vi "APC_9049_TS10ms_loop.vi"() -> ()   [LabVIEW 2020]
doc: "This example demonstrates the procedure required to apply different NI-DAQmx Custom Scales to each virtual channel in a task. A DAQmx Task Property Node (Functions >> NI Measurements >> DAQmx - Data Acquisition >> DAQmx Advanced Task Options) is used to obtain the task's virtual channels. A DAQmx Channel Property Node (Functions >> NI Measurements >> DAQmx - Data Acquisition) is then used to set the custom scale for each virtual channel in the task.\n\nThe \"DAQmx Create Scale\" VI creates a custom scale for each channel in the channel list. *Note, make sure your Minimum and Maximum channel parameters are consistent with the range the scale will create."
uses:
  <vilib>/Platform/TimedLoop/XDataNode/timing_clust.ctl
  <vilib>/Platform/TimedLoop/XDataNode/nitl_modes.ctl
  <vilib>/Platform/TimedLoop/XDataNode/wakeup.ctl
  controls/APC_ControlSettings.ctl
  controls/APC_PIDcontrolSettings.ctl
  <vilib>/FPGAPlugInAG/cRIO-9049/niLvFpga_Open_cRIO-9049.vi
  <vilib>/Powertrain Controls/Device Drivers/Tools/Real-Time/Interp1DTableRT.vi
  <vilib>/Utility/error.llb/Error Cluster From Error Code.vi
  <vilib>/rvi/errors/niLvFpgaAdjustHostInterfaceError.vi
  <vilib>/Powertrain Controls/Device Drivers/Tools/Real-Time/time2ticks.vi
  <vilib>/Powertrain Controls/Device Drivers/Tools/Real-Time/Offset2CAT.vi
  <vilib>/FPGAPlugInAG/cRIO-9049/niLvFpga_Close_cRIO-9049.vi
  <vilib>/Platform/TimedLoop/XDataNode/XDataNode.xnode
  <vilib>/rvi/interface/nirviOpenFPGA/nirviOpenFPGA.xnode
  FPGA Bitfiles/nobleapcmulticyl_FPGATarget4_APC9049FPGAmain_30BIM05nubg.lvbitx
  APC_9049_FPGA_main.vi
  <vilib>/rvi/interface/nirviReadWriteControl/nirviReadWriteControl.xnode
  <vilib>/rvi/interface/nirviCloseFPGA/nirviCloseFPGA.xnode
  <vilib>/Platform/TimedLoop/XDataNode/XDNodeRunTimeDep.lvlib
  NiFpgaLv.dll
panel:
  in  "Must Use Cam & Z":bool
  out "FPGA Heartbeat":bool
  in  "manual SA [CADBTDC]":dbl
  in  "manual INJ settings":T1={"Window_Start (DBTDC)"=90.0, "Window_End (DBTDC)"=-30.0, "PilotEnable"=FALSE, "PilotDuration (msec)"=0.0, "PilotAdvance (msec)"=0.0, "PreEnable"=FALSE, "PreDuration (msec)"=0.0, "PreAdvance (msec)"=0.0, "MainEnable"=FALSE, "MainDuration (msec)"=0.0, "MainSOI (DBTDC)"=0.0, "AfterEnable"=FALSE, "AfterDuration (msec)"=0.0, "AfterDelay (msec)"=0.0, "PostEnable"=FALSE, "PostDuration (msec)"=0.0, "PostDelay (msec)"=0.0}
  out "SA [CADBTDC]":dbl format="%.2f"
  in  "Override PC settings":bool
  in  "manual spark enable":bool[](array[boolean])
  in  "manual Injection enable":bool[](array[boolean])
  out "DI_Data Mod6":T2={"ModulePresent"=TRUE, "LVSense"=133, "HVSense"=23, "HVSense2"=1, "TempSense"=33, "Fault1"=126, "Fault2"=0, "OLIntegrator"=0, "HardwareRev"=70, "FirmwareRev"=5}
  in  "PFI0 mode":u8
  out "SparkControl_Out":T3
  in  "1/2 Z pulse":bool=TRUE
  out "toggle TDC":bool
  out "Finished Late? [i-1]":bool
  out "PlsGen_Config_Out":T4={"Channel Enable"=TRUE, "Seq_Start"=10800, "Seq_End"=15600, "Enable_Inj1"=FALSE, "Duration_Inj1"=0, "Timing_Inj1"=0, "Enable_Inj2"=FALSE, "Duration_Inj2"=0, "Timing_Inj2"=0, "Enable_Inj3"=TRUE, "Duration_Inj3"=160000, "Timing_Inj3"=14880, "Enable_Inj4"=FALSE, "Duration_Inj4"=0, "Timing_Inj4"=0, "Enable_Inj5"=FALSE, "Duration_Inj5"=0, "Timing_Inj5"=0}
  out "DI_Data_Mod5":T2={"ModulePresent"=TRUE, "LVSense"=133, "HVSense"=23, "HVSense2"=1, "TempSense"=33, "Fault1"=126, "Fault2"=0, "OLIntegrator"=0, "HardwareRev"=70, "FirmwareRev"=5}
  out "loop time [ms]":u32=10
  out "Speed (RPM)":sgl
  in  "Mod4/DIO7":bool
  in  "Mod4/DIO6":bool
  in  "Mod3/DIO7":bool
  in  "Mod3/DIO6":bool
  in  "Mod3/DIO5":bool
  in  "Mod3/DIO4":bool
  out "InjectionEnable":bool[](array[boolean])=[TRUE, TRUE, TRUE, TRUE, TRUE, TRUE]
  in  "Manual Clear Sync Errors":bool
  out "SparkEnable":bool[](array[boolean])=[TRUE, TRUE, TRUE, TRUE, TRUE, TRUE]
  in  "CutoffPosition (DBTDC)":sgl=-60.0
  out "PlsGen_Time_Config_In":T1={"Window_Start (DBTDC)"=90.0, "Window_End (DBTDC)"=-30.0, "PilotEnable"=FALSE, "PilotDuration (msec)"=0.0, "PilotAdvance (msec)"=0.0, "PreEnable"=FALSE, "PreDuration (msec)"=0.0, "PreAdvance (msec)"=0.0, "MainEnable"=TRUE, "MainDuration (msec)"=4.0, "MainSOI (DBTDC)"=-12.0, "AfterEnable"=FALSE, "AfterDuration (msec)"=0.0, "AfterDelay (msec)"=0.0, "PostEnable"=FALSE, "PostDuration (msec)"=0.0, "PostDelay (msec)"=0.0}
  in  "IPhaseArrayIn":T5(array[cluster])=[{"DriveSrc"=TRUE, "IUpper (A)"=11.0, "ILower (A)"=6.84, "Dur (msec)"=0.35}, {"DriveSrc"=FALSE, "IUpper (A)"=8.0, "ILower (A)"=6.84, "Dur (msec)"=0.25}, {"DriveSrc"=FALSE, "IUpper (A)"=3.9, "ILower (A)"=2.7, "Dur (msec)"=0.0}, {"DriveSrc"=FALSE, "IUpper (A)"=0.0, "ILower (A)"=0.0, "Dur (msec)"=0.0}, {"DriveSrc"=FALSE, "IUpper (A)"=0.0, "ILower (A)"=0.0, "Dur (msec)"=0.0}, {"DriveSrc"=FALSE, "IUpper (A)"=0.0, "ILower (A)"=0.0, "Dur (msec)"=0.0}, {"DriveSrc"=FALSE, "IUpper (A)"=0.0, "ILower (A)"=0.0, "Dur (msec)"=0.0}, {"DriveSrc"=FALSE, "IUpper (A)"=0.0, "ILower (A)"=0.0, "Dur (msec)"=0.0}]
  in  "DIControl":T6={"ModuleEnable"=TRUE, "HVEnable"=FALSE, "InjectEnable"=TRUE, "Phase1FirstPeakEnable"=FALSE, "PiezoEnable"=FALSE, "PiezoInvert"=FALSE, "OneShotSelect"=enum."DISABLED", "One Shot Time (msec)"=1.0, "OneShot"=FALSE, "Fault_ClrSig"=FALSE, "HVTarget (V)"=100.0, "Back Boost Time (msec)"=0.25, "DI Scope Trigger Event"=0, "DI Scope Channel 2"=0} {"DI Scope Trigger Event" items=["INJECTION PULSE", "POWER SUPPLY ENABLED"]; "DI Scope Channel 2" items=["INTERNAL HIGH VOLTAGE", "EXTERNAL HIGH VOLTAGE", "BATTERY VOLTAGE"]}
  in  "EPTControl":T7={"NumberOfCrankTeeth"=3600, "Stroke (FALSE=2, TRUE=4)"=TRUE, "CrankStallPeriod"=5000000, "CrankCountStart"=3600, "PeriodAccumCount"=3600, "SyncEnable"=TRUE, "SimEnable"=FALSE, "MissedCrankFlagClr"=FALSE, "MissedCamFlagClr"=FALSE, "SimPeriod"=500, "WatchdogIn"=FALSE}
  out "EPTData":T8={"CrankSigOS"=FALSE, "CrankStalled"=FALSE, "SyncStopped"=FALSE, "MissedCrankFlag"=FALSE, "MissedCamFlag"=FALSE, "Period"=863, "PeriodAccum"=2084945, "CrankCount"=928, "CurrentPosition"=3712, "MAX_CAT"=28800}
  # "Override PC settings option disabled"
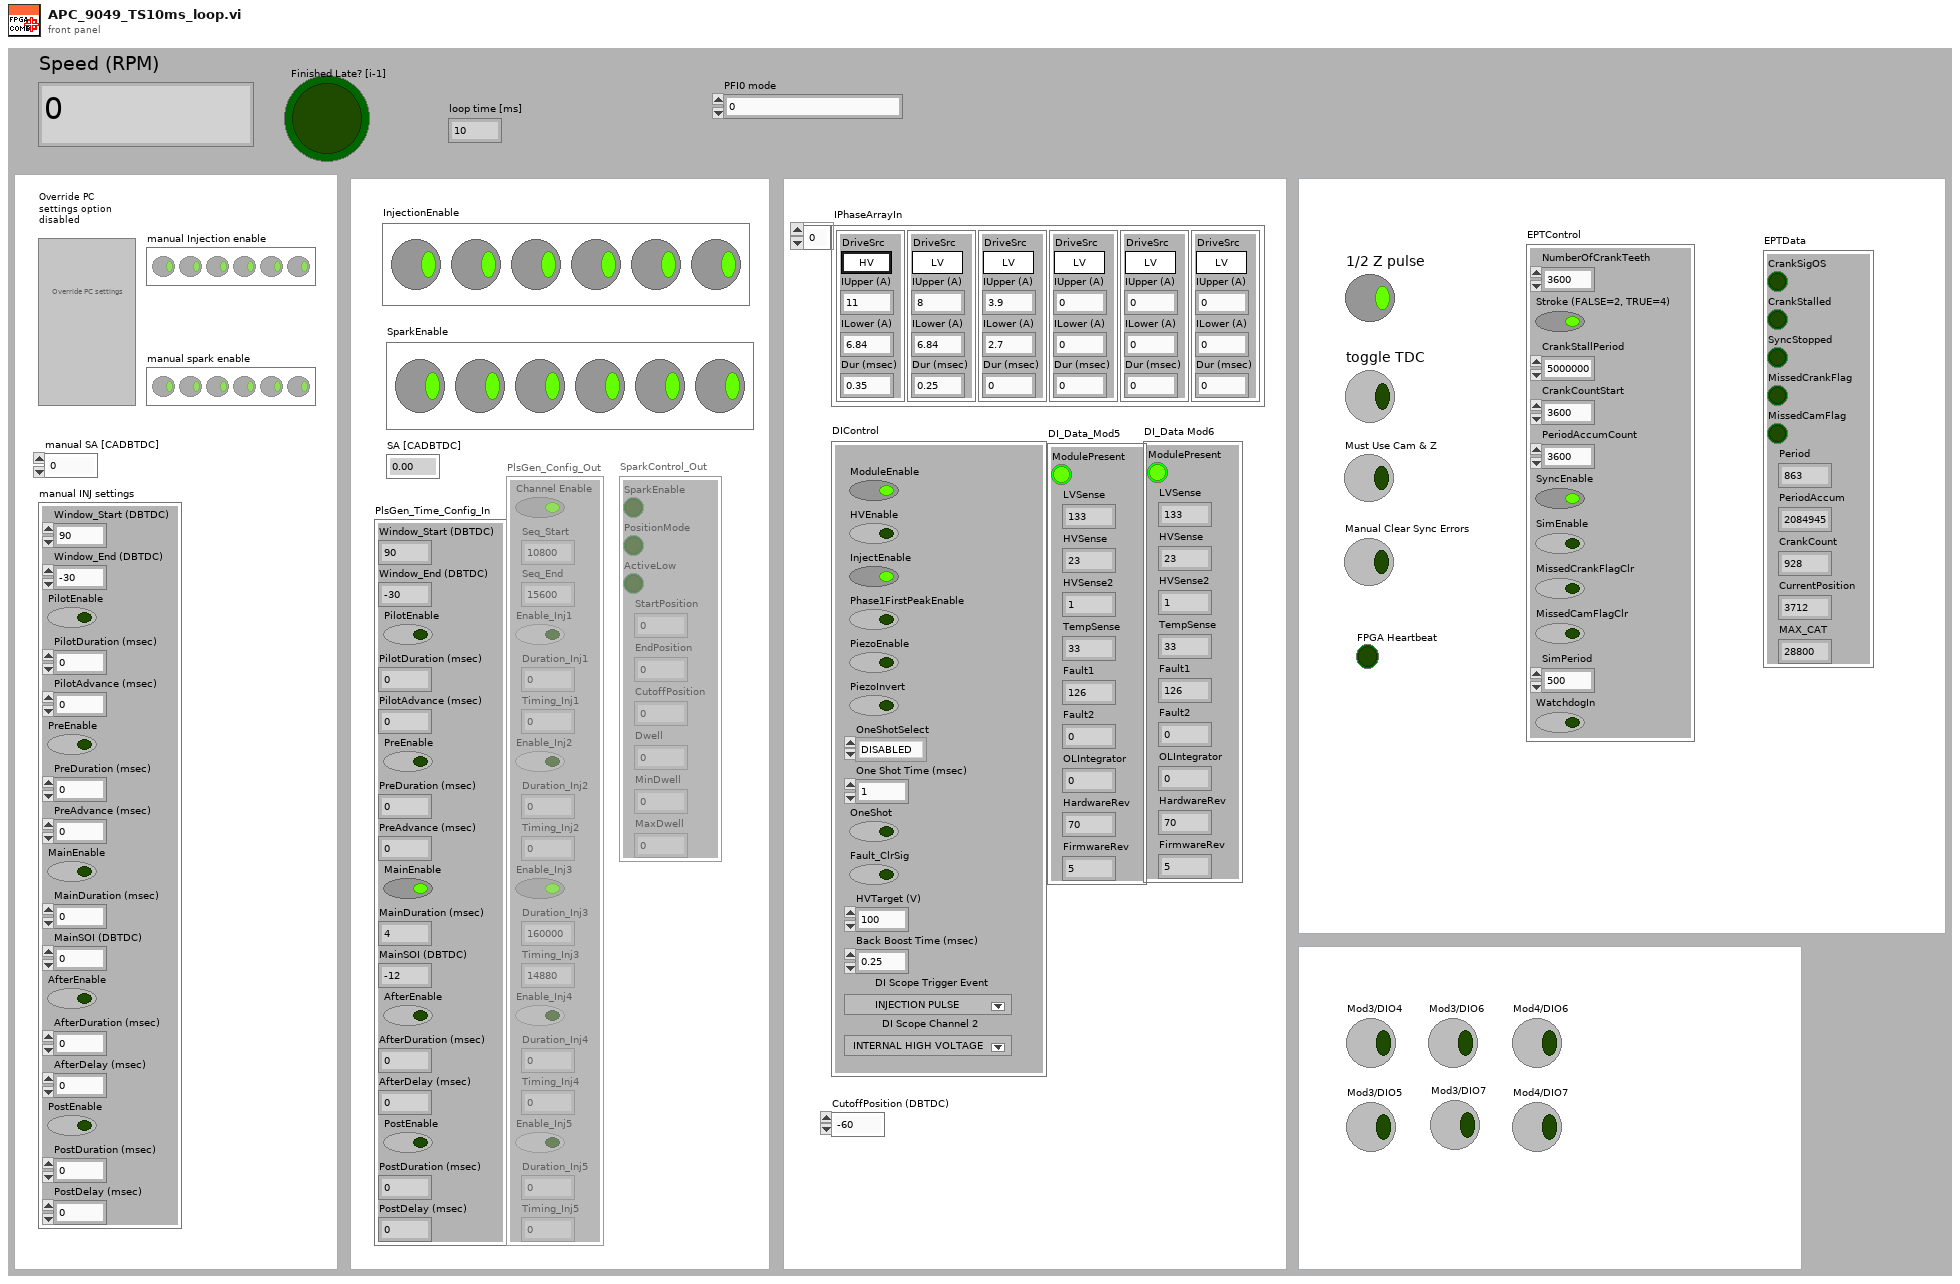
[diagram p1: front panel]
types:
  T1 = cluster{"Window_Start (DBTDC)":sgl, "Window_End (DBTDC)":sgl, "PilotEnable":bool, "PilotDuration (msec)":sgl, "PilotAdvance (msec)":sgl, "PreEnable":bool, "PreDuration (msec)":sgl, "PreAdvance (msec)":sgl, "MainEnable":bool, "MainDuration (msec)":sgl, "MainSOI (DBTDC)":sgl, "AfterEnable":bool, "AfterDuration (msec)":sgl, "AfterDelay (msec)":sgl, "PostEnable":bool, "PostDuration (msec)":sgl, "PostDelay (msec)":sgl}
  T2 = cluster{"ModulePresent":bool, "LVSense":u8, "HVSense":u8, "HVSense2":u8, "TempSense":i8, "Fault1":u8, "Fault2":u8, "OLIntegrator":u32, "HardwareRev":u8, "FirmwareRev":u8}
  T3 = cluster{"SparkEnable":bool, "PositionMode":bool, "ActiveLow":bool, "StartPosition":u16, "EndPosition":u16, "CutoffPosition":u16, "Dwell":u32, "MinDwell":u32, "MaxDwell":u32}
  T4 = cluster{"Channel Enable":bool, "Seq_Start":u16, "Seq_End":u16, "Enable_Inj1":bool, "Duration_Inj1":u32, "Timing_Inj1":u32, "Enable_Inj2":bool, "Duration_Inj2":u32, "Timing_Inj2":u32, "Enable_Inj3":bool, "Duration_Inj3":u32, "Timing_Inj3":u16, "Enable_Inj4":bool, "Duration_Inj4":u32, "Timing_Inj4":u32, "Enable_Inj5":bool, "Duration_Inj5":u32, "Timing_Inj5":u32}
  T5 = cluster{"DriveSrc":bool, "IUpper (A)":sgl, "ILower (A)":sgl, "Dur (msec)":sgl}[]
  T6 = cluster{"ModuleEnable":bool, "HVEnable":bool, "InjectEnable":bool, "Phase1FirstPeakEnable":bool, "PiezoEnable":bool, "PiezoInvert":bool, "OneShotSelect":enum8{"DISABLED", "CHAN 1", "CHAN 2", "CHAN 3"}, "One Shot Time (msec)":sgl, "OneShot":bool, "Fault_ClrSig":bool, "HVTarget (V)":sgl, "Back Boost Time (msec)":sgl, "DI Scope Trigger Event":u16, "DI Scope Channel 2":u16}
  T7 = cluster{"NumberOfCrankTeeth":u16, "Stroke (FALSE=2, TRUE=4)":bool, "CrankStallPeriod":u32, "CrankCountStart":u16, "PeriodAccumCount":u16, "SyncEnable":bool, "SimEnable":bool, "MissedCrankFlagClr":bool, "MissedCamFlagClr":bool, "SimPeriod":u32, "WatchdogIn":bool}
  T8 = cluster{"CrankSigOS":bool, "CrankStalled":bool, "SyncStopped":bool, "MissedCrankFlag":bool, "MissedCamFlag":bool, "Period":u32, "PeriodAccum":u32, "CrankCount":u16, "CurrentPosition":u16, "MAX_CAT":u16}
  T9 = typedef "XDNodeRunTimeDep.lvlib/timing_clust.ctl" = cluster{"Expected End [f-1]":u64, "Actual End [f-1]":u64, "Finished Late? [f-1]":bool, "Expected End [i-1]":u64, "Actual End [i-1]":u64, "Finished Late? [i-1]":bool, "Expected Start [i]":u64, "Actual Start [i]":u64, "Expected Start [f]":u64, "Actual Start [f]":u64, "Source Name":string, "Structure Name":string, "Period":i64, "Deadline":i64, "Offset":i64, "Start":i64, "Priority":i32, "Timeout":i32, "Mode":T10, "Wakeup Reason":T11, "Error":errorcluster, "Source Type":string, "Secondary Source Type":string, "Global End Time":u64, "Global Start Time":u64, "Frame Duration":u64, "Iteration Duration":u64, "Assigned CPU":i32, "I/O Scan Engine Mode":u32}
  T10 = typedef "XDNodeRunTimeDep.lvlib/nitl_modes.ctl" = enum32{"No Change", "Process missed periods, maintain original phase", "Discard missed periods, maintain original phase", "Process missed periods, ignore original phase", "Discard missed periods, ignore original phase"}
  T11 = typedef "XDNodeRunTimeDep.lvlib/wakeup.ctl" = enum32{"Normal", "Aborted", "Asynchronous wakeup", "Timing source error", "Timed loop error", "Timeout"}
  T12 = typedef "APC_ControlSettings.ctl" = cluster{"Spark advance [CADBTDC]":dbl, "Pref":dbl, "O2ref":dbl, "DI advance [CADBTDC]":dbl, "DI duration [ms] ":dbl, "CO2ref":dbl, "PFI duration [ms]":dbl, "IMEP ref":dbl, "Speed ref":dbl, "IGN enable":bool, "DI enable":bool, "CL PFI\n lambda":bool, "CL PFI\nIMEP":bool, "Activate\ncylinder":bool[], "Force idling":bool, "Force motoring":bool, "ETP resync":bool, "Requested mode":i8, "Clear Sync Errors":bool, "toggle TDC":bool, "l ref":dbl, "PID control references":T13, "CA50setpoint [CADATDC]":dbl, "CA50 control":bool, "Knock control":bool, "CLEAR EMERGENCY STOP":bool, "EMERGENCY STOP":bool}
  T13 = typedef "APC_PIDcontrolSettings.ctl" = cluster{"NG":bool, "Ar":bool, "O2":bool, "Intake vent":bool, "Cross vent":bool, "Exhaust vent":bool, "NG control mode":u8, "NG-FC-001-REF":dbl, "WF-OA-002-REF":dbl, "IMEP-REF":dbl, "Nm-REF":dbl, "Ar control mode":u8, "AR-PC-002-REF":dbl, "WF-PT-004-REF":dbl, "O2 control mode":u8, "O2-FC-001-REF":dbl, "WF-OA-001-REF":dbl, "Tcoolant control  mode":u8, "EC-FC-001-REF":dbl, "EC-TT-001-REF":dbl, "Texh control mode":u8, "SW-FC-004-REF":dbl, "SW-FT-002-REF":dbl, "WF-TT-004-REF":dbl, "Toil control mode":u8, "SW-FC-009-REF":dbl, "SW-FT-004-REF":dbl, "EO-TT-001-REF":dbl, "AIC201_CO2_ConcTarget":dbl, "O2_FF_NG":bool, "Dyno control mode":u8, "Membrane control mode":u8, "AR-FT-001-REF":dbl, "MTR modbus floats":sgl[], "MTR modbus u16":u16[], "MTR HB":bool, "PC_HB":bool, "EMERGENCY STOP":bool}
  T14 = cluster{"ModuleEnable":bool, "WatchdogIn":bool, "OneShotSelect":enum8{"DISABLED", "CHAN 1", "CHAN 2", "CHAN 3"}, "OneShotTime":u32, "OneShot":bool, "Control":u8, "Control2":u8, "HostMode":u8, "HostCommand":u32, "HVTarget":u8, "BackBoostTime":u8, "Fault_ClrSig":bool}
  T15 = cluster{"IPhaseDrive (TRUE=HV, FALSE=LV)":bool, "IPhaseCurrentUpper":u16, "IPhaseCurrentLower":u16, "IPhaseDuration":u16}[]
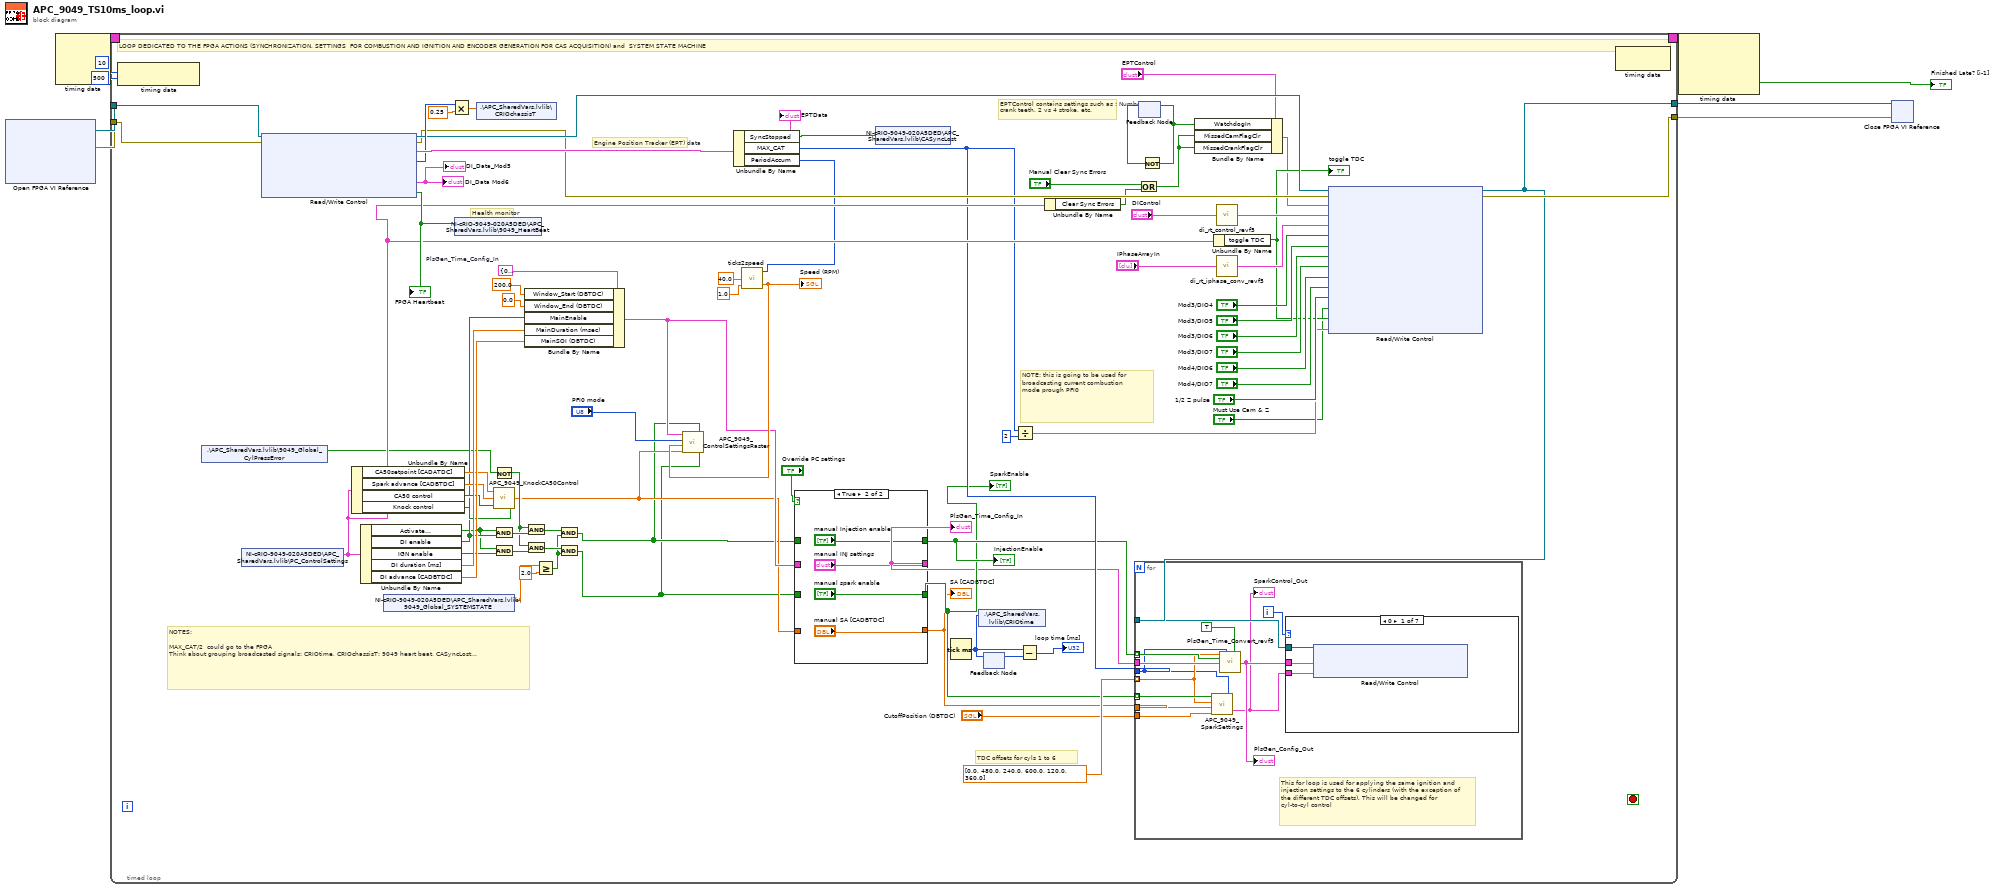
[diagram p0: block diagram]
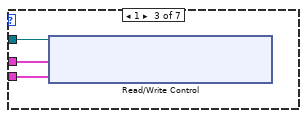
[diagram p4: hidden frame]
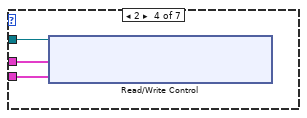
[diagram p5: hidden frame]
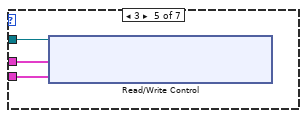
[diagram p6: hidden frame]
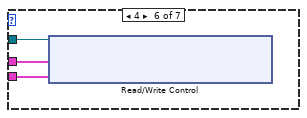
[diagram p7: hidden frame]
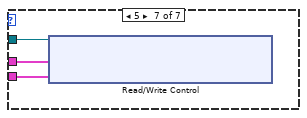
[diagram p8: hidden frame]
diagram:
  n1 = xnode "Open FPGA VI Reference"() -> ("FPGA VI Reference Out"=w5:refnum<k20>, "error out"=w4:errorcluster)  [unwired: 2 in]
  n2 = node-c288(i64 10 ("Period"), 500 ("Priority")) -> (w9:T9)  [unwired: 1 in]
  n3 = timed-loop {
    timing: w9 -> [_]
    timing-out: [_] -> w8
    tunnel: [w70] -> w2
    tunnel: w5 -> [w78]
    tunnel: w4 -> [w77]
    tunnel: [w76] -> w1
    stop <- _ stop-if-true
    w57 = T1 {"Window_Start (DBTDC)"=0.0, "Window_End (DBTDC)"=0.0, "PilotEnable"=FALSE, "PilotDuration (msec)"=0.0, "PilotAdvance (msec)"=0.0, "PreEnable"=FALSE, "PreDuration (msec)"=0.0, "PreAdvance (msec)"=0.0, "MainEnable"=FALSE, "MainDuration (msec)"=0.0, "MainSOI (DBTDC)"=0.0, "AfterEnable"=FALSE, "AfterDuration (msec)"=0.0, "AfterDelay (msec)"=0.0, "PostEnable"=FALSE, "PostDuration (msec)"=0.0, "PostDelay (msec)"=0.0}  # PlsGen_Time_Config_In
    # "EPTControl contains settings such as : Number of crank teeth, 2 vs 4 stroke, etc."
    # "Health monitor"
    # "Engine Position Tracker (EPT) data"
    # "NOTE: this is going to be used for broadcasting current combustion mode prough PFI0"
    # "NOTES:\n\nMAX_CAT/2  could go to the FPGA\nThink about grouping broadcasted signals: CRIOtime, CRIOchassisT: 9049 heart beat, CASyncLost..."
    # "TDC offsets for cyls 1 to 6"
    # "LOOP DEDICATED TO THE FPGA ACTIONS (SYNCHRONIZATION, SETTINGS  FOR COMBUSTION AND IGNITION AND ENCODER GENERATION FOR CAS ACQUISITION) and  SYSTEM STATE MACHINE"
    n4 = node-c288() -> ()  [unwired: 1 in, 1 out]
    n5 = shared-variable ".\\APC_SharedVars.lvlib\\9049_Global_CylPressError"() -> (w28:bool)  [unwired: 1 in, 1 out]
    n6 = shared-variable "NI-cRIO-9049-020A5DED\\APC_SharedVars.lvlib\\PC_ControlSettings"() -> (w42:T12)  [unwired: 1 in, 1 out]
    n7 = xnode "Read/Write Control"("FPGA VI Reference In"=w78, "error in"=w77) -> ("FPGA VI Reference Out"=w80:refnum<k20>, "error out"=w75:errorcluster, "EPTData"=w85:T8, "Chassis Temp Raw (x4 C)"=w82:i16, "DI_Data_Mod6"=→"DI_Data_Mod5" →"DI_Data Mod6":T2, "FPGA Heartbeat"=w48:bool)  [unwired: 1 out]
    "EPTData" <- w85
    "FPGA Heartbeat" <- w48
    n8 = Unbundle By Name(w42) -> ("CA50setpoint [CADATDC]"=w44:dbl, "Spark advance [CADBTDC]"=w43:dbl, "CA50 control"=w46:bool, "Knock control"=w45:bool)
    n9 = Unbundle By Name(w42) -> ("Activate\ncylinder"=w40:bool[], "DI enable"=w41:bool, "IGN enable"=w39:bool, "DI duration [ms]"=w54:dbl, "DI advance [CADBTDC]"=w53:dbl)
    n10 = shared-variable "NI-cRIO-9049-020A5DED\\APC_SharedVars.lvlib\\9049_Global_SYSTEMSTATE"() -> (w26:dbl)  [unwired: 1 in, 1 out]
    n11 = Multiply(x=w82, y=0.25) -> (x*y=w79:dbl)
    n12 = shared-variable "NI-cRIO-9049-020A5DED\\APC_SharedVars.lvlib\\9049_HeartBeat"(w48) -> ()  [unwired: 1 in, 1 out]
    n13 = shared-variable ".\\APC_SharedVars.lvlib\\CRIOchassisT"(w79) -> ()  [unwired: 1 in, 1 out]
    n14 = Not(x=w28) -> (.not. x?=w27:bool)
    n15 = call "APC_9049_KnockCA50Control.vi"("Knock control?"=w45, "CA50 control?"=w46, "Manual SA [CADBTDC]"=w43, "CA50setpoint [CADATDC]"=w44) -> ("SA [CADBTDC]"=w17:dbl)  [unwired: 1 in]
    n16 = And(x=w40, y=w41) -> (x .and. y?=w30:bool[])
    n17 = And(x=w40, y=w39) -> (x .and. y?=w29:bool[])
    n18 = Bundle By Name(cluster=w57, "Window_Start (DBTDC)"=sgl 200.0, "Window_End (DBTDC)"=sgl 0.0, "MainEnable"=w41, "MainDuration (msec)"=w54, "MainSOI (DBTDC)"=w53) -> (w19:T1)
    n19 = And(x=w27, y=w30) -> (x .and. y?=w24:bool[])
    n20 = And(x=w27, y=w29) -> (x .and. y?=w23:bool[])
    n21 = Greater Or Equal?(x=w26, y=2.0) -> (x >= y?=w22:bool)
    n22 = And(x=w24, y=w22) -> (x .and. y?=w15:bool[])
    n23 = And(x=w23, y=w22) -> (x .and. y?=w14:bool[])
    n24 = Unbundle By Name(w85) -> ("SyncStopped"=w38:bool, "MAX_CAT"=w36:u16, "PeriodAccum"=w37:u32)
    n25 = call <vilib>:"ticks2speed.vi"("PulsesPerRotation"=sgl 1.0, "Clock Frequency (MHz, 40)"=sgl 40.0, "Period (ticks)"=w37) -> ("Speed (RPM)"=w58:sgl)  [unwired: 1 out]
    "Speed (RPM)" <- w58
    n26 = call "APC_9049_ControlSettingsRaster.vi"("SparkEnable"=w14, "InjectionEnable"=w15, "SparkTiming (DBTDC) loc"=w17, "Speed (RPM)"=w58, "9049 STATE"="PFI0 mode", "PlsGen_Time_Config_In"=w19) -> ()
    n27 = case shown="True" "Override PC settings" {
      tunnel: [w88 "manual Injection enable"] -> w21
      tunnel: [w87 "manual spark enable"] -> w20
      tunnel: [w89 "manual SA [CADBTDC]"] -> w16
      tunnel: [w90 "manual INJ settings"] -> w18
      tunnel: w19 -> [w90 _]
      tunnel: w17 -> [w89 _]
      tunnel: w15 -> [w88 _]
      tunnel: w14 -> [w87 _]
      frame False {
      }
      frame True {
      }
    }
    "PlsGen_Time_Config_In" <- w18
    "SparkEnable" <- w20
    "InjectionEnable" <- w21
    "SA [CADBTDC]" <- w16
    n28 = shared-variable "NI-cRIO-9049-020A5DED\\APC_SharedVars.lvlib\\CASyncLost"(w38) -> ()  [unwired: 1 in, 1 out]
    n29 = Tick Count (ms)() -> (millisecond timer value=w63:u32)
    n30 = shared-variable ".\\APC_SharedVars.lvlib\\CRIOtime"(w63) -> ()  [unwired: 1 in, 1 out]
    n31 = feedback #1() -> (w62:u32)  [unwired: 1 in]
    n32 = feedback-in #1(w63) -> ()
    n33 = Divide(x=w36, y=u16 2) -> (x/y=w49:dbl)
    n34 = Subtract(x=w63, y=w62) -> (x-y=→"loop time [ms]":u32)
    n35 = Unbundle By Name(w42) -> ("Clear Sync Errors"=w34:bool)
    n36 = Or(x="Manual Clear Sync Errors", y=w34) -> (x .or. y?=w32:bool)
    n37 = feedback #2() -> (w86:bool)  [unwired: 1 in]
    n38 = Not(x=w86) -> (.not. x?=w60:bool)
    n39 = feedback-in #2(w60) -> ()
    n40 = Bundle By Name(cluster="EPTControl", "WatchdogIn"=w60, "MissedCamFlagClr"=w32, "MissedCrankFlagClr"=w32) -> (w11:T7)
    n41 = Unbundle By Name(w42) -> ("toggle TDC"=w51:bool)
    "toggle TDC" <- w51
    n42 = call <vilib>:"di_rt_control_revf5.vi"("DIControl"="DIControl") -> ("DIControlToFPGA"=w72:T14)  [unwired: 4 in]
    n43 = call <vilib>:"di_rt_iphase_conv_revf5.vi"("IPhaseArrayIn"="IPhaseArrayIn") -> ("IPhaseArrayOut"=w71:T15)
    n44 = xnode "Read/Write Control"("FPGA VI Reference In"=w80, "error in"=w75, "EPTControl"=w11, "DI_Control"=w72, "DI_IPhaseInterface"=w71, "Mod3/DIO4"="Mod3/DIO4", "Mod3/DIO5"="Mod3/DIO5", "Mod3/DIO6"="Mod3/DIO6", "Mod3/DIO7"="Mod3/DIO7", "Mod4/DIO6"="Mod4/DIO6", "Mod4/DIO7"="Mod4/DIO7", "1/2 Z pulse"="1/2 Z pulse", "Must Use Cam & Z"="Must Use Cam & Z", "toggle TDC"=w51, "TRIG1_offset_ticks"=w49) -> ("FPGA VI Reference Out"=w70:refnum<k20>, "error out"=w76:errorcluster)
    n45 = for {
      tunnel: w18 -> [w106]
      tunnel: w20 -> [w100] mode=indexing
      tunnel: dbl[] [0.0, 480.0, 240.0, 600.0, 120.0, 360.0] -> [w99] mode=indexing
      tunnel: w16 -> [w98]
      tunnel: "CutoffPosition (DBTDC)" -> [w97]
      tunnel: w70 -> [w102]
      tunnel: w21 -> [w101] mode=indexing
      tunnel: w36 -> [w95]
      i -> [w103]
      # "This for loop is used for applying the same ignition and injection settings to the 6 cylinders (with the exception of the different TDC offsets). This will be changed for cyl-to-cyl control"
      n46 = call "APC_9049_SparkSettings.vi"("MAX_CAT"=w95, "CutoffPosition (DBTDC)"=w97, "SparkTiming (DBTDC) loc"=w98, "TDC (Absolute CAD)"=w99, "SparkEnable"=w100) -> ("SparkControl"=w96:T3)
      "SparkControl_Out" <- w96
      n47 = call <vilib>:"PlsGen_Time_Convert_revf5.vi"("TDC (Absolute CAD)"=w99, "MAX_CAT"=w95, "Stroke (FALSE=2, TRUE=4)"=TRUE, "Channel Enable"=w101, "PlsGen_Time_Config_In"=w106) -> ("PlsGen_Config_Out"=w105:T4)  [unwired: 10 in]
      "PlsGen_Config_Out" <- w105
      n48 = case shown="0" w103 {
        tunnel: w105 -> [w109 _ w112 w115 w118 w121 w124]
        tunnel: w96 -> [w108 _ w111 w114 w117 w120 w123]
        tunnel: w102 -> [w107 _ w110 w113 w116 w119 w122]
        frame 0 {
          n49 = xnode "Read/Write Control"("FPGA VI Reference In"=w107, "DI 1"=w109, "Spark 1"=w108) -> ()  [unwired: 1 in, 2 out]
        }
        frame 6, Default {
        }
        frame 1 {
          n50 = xnode "Read/Write Control"("FPGA VI Reference In"=w110, "DI 2"=w112, "Spark 2"=w111) -> ()  [unwired: 1 in, 2 out]
        }
        frame 2 {
          n51 = xnode "Read/Write Control"("FPGA VI Reference In"=w113, "DI 3"=w115, "Spark 3"=w114) -> ()  [unwired: 1 in, 2 out]
        }
        frame 3 {
          n52 = xnode "Read/Write Control"("FPGA VI Reference In"=w116, "DI 4"=w118, "Spark 4"=w117) -> ()  [unwired: 1 in, 2 out]
        }
        frame 4 {
          n53 = xnode "Read/Write Control"("FPGA VI Reference In"=w119, "DI 5"=w121, "Spark 5"=w120) -> ()  [unwired: 1 in, 2 out]
        }
        frame 5 {
          n54 = xnode "Read/Write Control"("FPGA VI Reference In"=w122, "DI 6"=w124, "Spark 6"=w123) -> ()  [unwired: 1 in, 2 out]
        }
      }
    }
    n55 = node-c288() -> ()  [unwired: 1 in, 1 out]
  }
  n56 = node-c288(w8) -> (→"Finished Late? [i-1]":bool)  [unwired: 3 out]
  n57 = xnode "Close FPGA VI Reference"("FPGA VI Reference In"=w2, "error in"=w1) -> ()  [unwired: 1 out]
